vi "Mock Process Error.vi"(8 "error in (no error)":errorcluster, 10 "Mock Error":errorcluster, 11 "Mock Process in":refnum<class "Mock Process.lvclass">) -> (0 "error out":errorcluster, 3 "Mock Process out":refnum<class "Mock Process.lvclass">)   [LabVIEW 2020, in "Mock Process.lvclass"]
uses:
  Mock Process.lvclass
  Framework/Process/Process.lvclass
  C:/Users/anton/Documents/GitHub/Triarc-Framework/source/Framework/Process/Process.lvclass
  C:/Users/anton/Documents/GitHub/Triarc-Framework/source/Framework/Base/Base.lvclass
  C:/Users/anton/Documents/GitHub/Triarc-Framework/source/Framework/Configuration File/Configuration File.lvclass
  C:/Users/anton/Documents/GitHub/Triarc-Framework/source/Framework/Configuration/Configuration.lvclass
  C:/Users/anton/Documents/GitHub/Triarc-Framework/source/Framework/Error Handler Interface/Error Handler Interface.lvclass
  C:/Users/anton/Documents/GitHub/Triarc-Framework/source/Framework/Logging/Logging.lvclass
  C:/Users/anton/Documents/GitHub/Triarc-Framework/source/Framework Test/Mock Process/Mock Process.lvclass
  C:/Users/anton/Documents/GitHub/Triarc-Framework/source/Framework/Async Handler/Async Handler.lvclass
  C:/Users/anton/Documents/GitHub/Triarc-Framework/source/Framework/Helper Loop/Helper Loop.lvclass
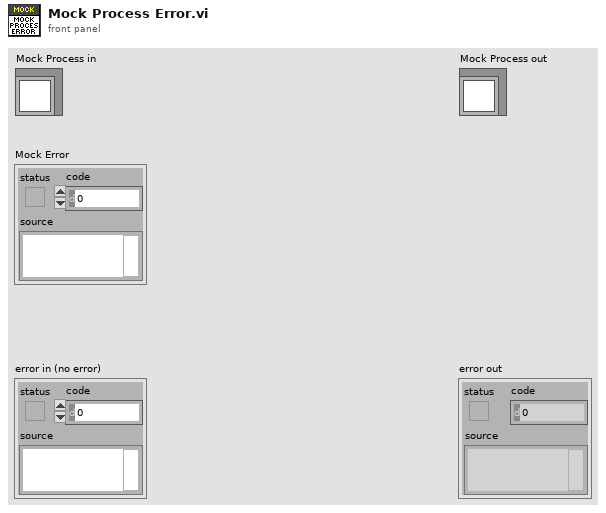
[diagram p1: front panel]
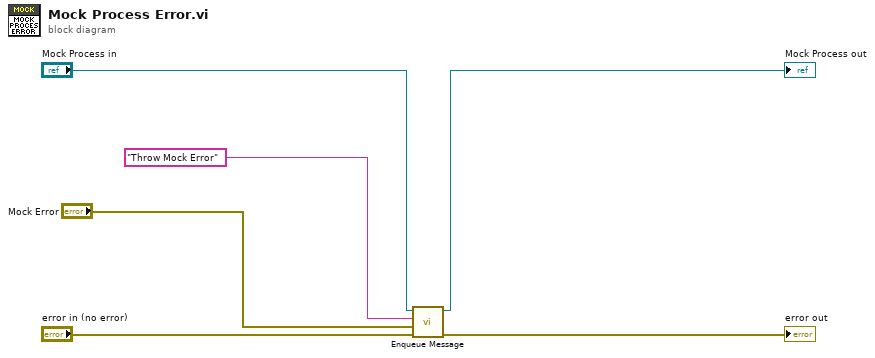
[diagram p0: block diagram]
diagram:
  n1 = call "Enqueue Message.vi"("error in (no error)"="error in (no error)", "Message Data"="Mock Error", "Message"="Throw Mock Error", "Process In"="Mock Process in") -> ("error out"=→"error out":errorcluster, "Process Out"=→"Mock Process out":refnum<class "Mock Process.lvclass">)  [unwired: 6 in]
